vi "solar Menu (Handle).vi"(5 "Target":string, 6 "Is SOLAR UI? (F)":bool, 7 "SOLAR Refnum":T1, 8 "error in (no error)":errorcluster, 9 "ItemTag":string, 10 "MenuRef":refnum<k9>, 11 "VIRef":refnum<vi>) -> (0 "error out":errorcluster)   [LabVIEW 2018]
doc: "This handles the menu selections for the target."
uses:
  <vilib>/Platform/browser.llb/Open URL in Default Browser (string).vi
  solar_ctl SOLAR UI Panes.ctl
  solar_ctl SOLAR Refnum.ctl
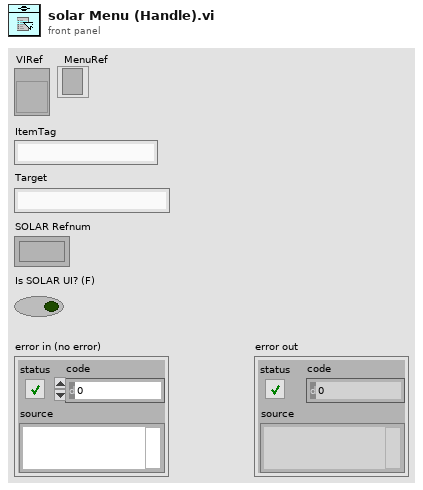
[diagram p1: front panel]
types:
  T1 = typedef "solar_ctl SOLAR Refnum.ctl" = refnum<k1>
  T2 = typedef "solar_ctl SOLAR Global.ctl" = cluster{"Targets":T3[], "AppDir":path, "solar.ini":path, "ConfigsDir":path, "CosmosDir":path, "LogsDir":path, "ExePath":path, "ExeVersion":string, "PartNum":string, "AppSetup":string, "Title":string, "Main.ini":path, "Temp.ini":path, "vSOLAR":string, "Splash.png":string, "SplashWait":i32, "SOLARUE":refnum<user-event>, "VoyagerRefnum":T4, "QTimerRefnum":T5}
  T3 = typedef "solar_ctl Target Global.ctl" = cluster{"Target":string, "Q":refnum<queue>, "UE":refnum<user-event>, "VI":refnum<vi>, "Menu":refnum<k9>, "Data":refnum<data-value>, "Attributes":variant}
  T4 = typedef "solar_voy_ctl Voyager Refnum.ctl" = refnum<k1>
  T5 = typedef "solar_qtimer_ctl Refnum.ctl" = refnum<k1>
  T6 = typedef "solar_ctl SOLAR UI Panes.ctl" = cluster{"Status":bool, "Emergency":bool, "Targets":bool}
  T7 = enum32{"invalid app kind", "Development System", "Run Time System", "Student Edition", "Embedded LabVIEW", "Evaluation", "Custom"}
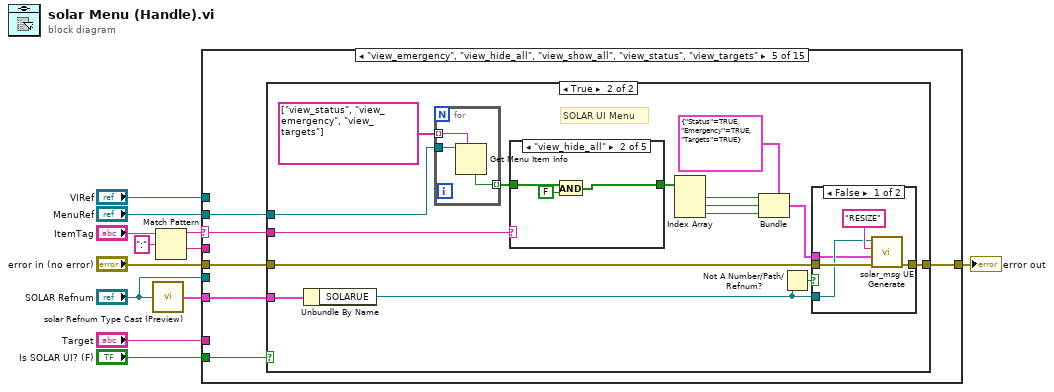
[diagram p0: block diagram]
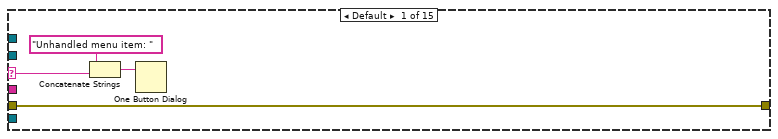
[diagram p2: hidden frame]
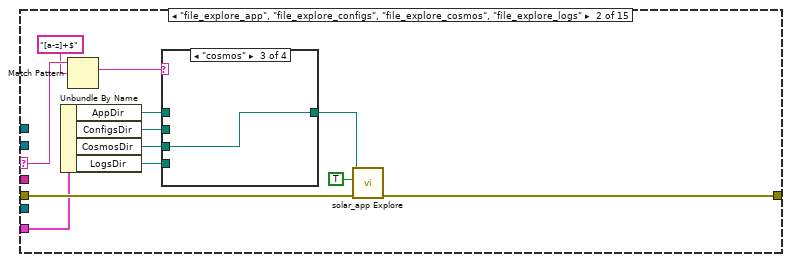
[diagram p3: hidden frame]
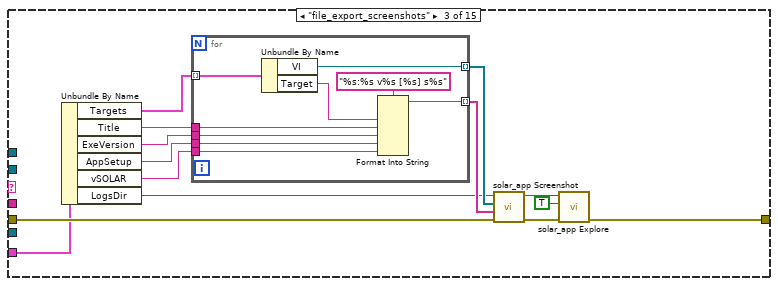
[diagram p7: hidden frame]
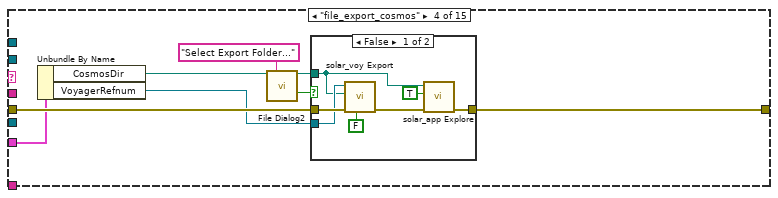
[diagram p8: hidden frame]
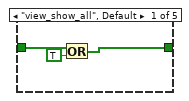
[diagram p11: hidden frame]
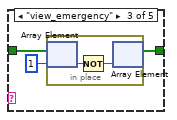
[diagram p12: hidden frame]
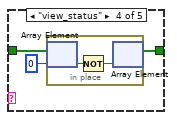
[diagram p13: hidden frame]
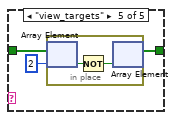
[diagram p14: hidden frame]
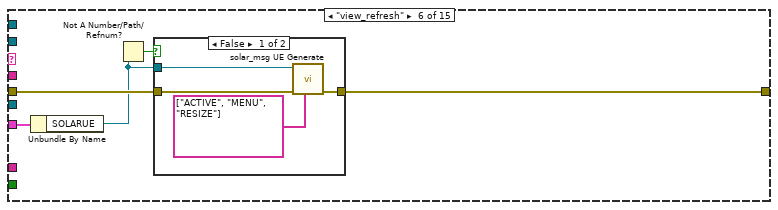
[diagram p16: hidden frame]
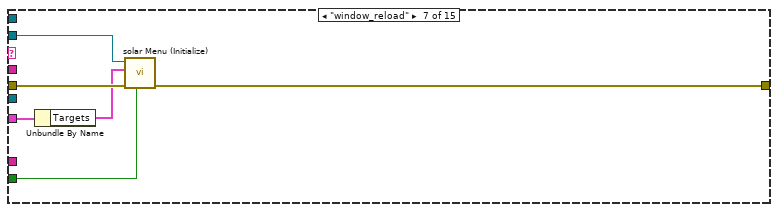
[diagram p18: hidden frame]
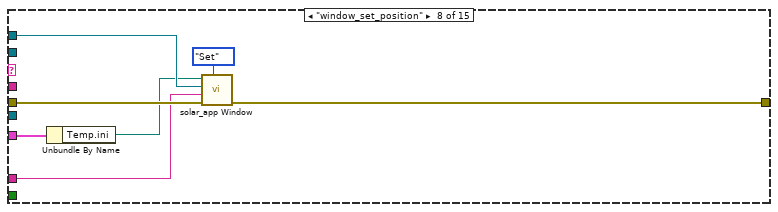
[diagram p19: hidden frame]
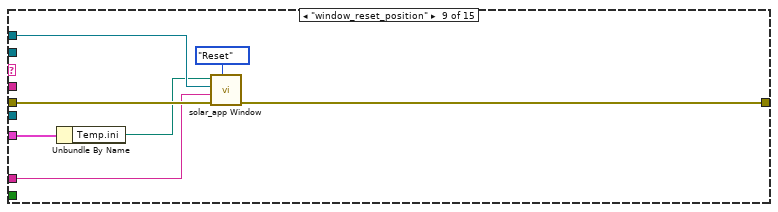
[diagram p20: hidden frame]
diagram:
  n1 = call "solar Refnum Type Cast (Preview).vi"("Refnum"="SOLAR Refnum") -> ("SOLAR"=w2:T2)  [unwired: 8 in]
  n2 = Match Pattern(string="ItemTag", regular expression=":") -> (before substring=w6:string, after substring=w5:string)  [unwired: 1 in, 2 out]
  n3 = case shown="\"view_emergency\", \"view_hide_all\", \"view_show_all\", \"view_status\", \"view_targets\"" w6 {
    selector: w6 -> [w15 w28 _ _ w73 _ _ _ _ _ _ _ _ _ _]
    tunnel: [w16 w24 w42 w63 w77 w128 w139 w143 w150 w157 w167 w185 w187 w211 w213] -> w12
    tunnel: "error in (no error)" -> [w16 w25 w46 w62 w76 w127 w137 w146 w153 w160 w168 w186 w188 w203 w214]
    tunnel: "VIRef" -> [_ _ _ _ _ _ _ w145 w152 w159 _ _ _ _ _]
    tunnel: "MenuRef" -> [_ _ _ _ w74 _ w138 _ _ _ _ _ _ _ _]
    tunnel: w5 -> [_ _ _ _ _ _ _ _ _ _ w166 w184 _ _ _]
    tunnel: "Is SOLAR UI? (F)" -> [_ _ _ _ w72 _ w135 _ _ _ _ _ _ _ _]
    tunnel: w2 -> [_ w21 w34 w57 w75 w125 w136 w141 w148 w155 w164 _ _ w202 _]
    tunnel: "Target" -> [_ _ _ _ _ _ _ w140 w147 w154 _ _ _ _ _]
    tunnel: "SOLAR Refnum" -> [_ _ _ _ _ _ _ _ _ _ _ w182 _ _ _]
    frame Default {
      n4 = Concatenate Strings("Unhandled menu item: ", w15) -> (w14:string)
      n5 = One Button Dialog(message=w14) -> ()  [unwired: 1 in, 1 out]
    }
    frame "file_explore_app", "file_explore_configs", "file_explore_cosmos", "file_explore_logs" {
      n6 = Unbundle By Name(w21) -> ("AppDir"=w17:path, "ConfigsDir"=w20:path, "CosmosDir"=w19:path, "LogsDir"=w18:path)
      n7 = Match Pattern(string=w28, regular expression="[a-z]+$") -> (match substring=w26:string)  [unwired: 1 in, 3 out]
      n8 = case shown="\"cosmos\"" w26 {
        tunnel: w20 -> [_ w30 _ _]
        tunnel: [w29 w30 w31 w32] -> w23
        tunnel: w19 -> [_ _ w31 _]
        tunnel: w18 -> [_ _ _ w32]
        tunnel: w17 -> [w29 _ _ _]
        frame "app", Default {
        }
        frame "configs" {
        }
        frame "cosmos" {
        }
        frame "logs" {
        }
      }
      n9 = call "solar_app Explore.vi"("error in (no error)"=w25, "Open Folder? (F)"=TRUE, "File or Folder Path"=w23) -> ("error out"=w24:errorcluster)  [unwired: 8 in]
    }
    frame "file_export_screenshots" {
      n10 = Unbundle By Name(w34) -> ("Targets"=w33:T3[], "Title"=w40:string, "ExeVersion"=w39:string, "AppSetup"=w38:string, "vSOLAR"=w37:string, "LogsDir"=w35:path)
      n11 = for {
        tunnel: [w55] -> w45 mode=indexing
        tunnel: w39 -> [w53]
        tunnel: w38 -> [w52]
        tunnel: w37 -> [w51]
        tunnel: w40 -> [w50]
        tunnel: [w48] -> w36 mode=indexing
        tunnel: w33 -> [w47] mode=indexing
        n12 = Unbundle By Name(w47) -> ("VI"=w48:refnum<vi>, "Target"=w49:string)
        n13 = Format Into String(format string="%s:%s v%s [%s] s%s", w49, w50, w53, w52, w51) -> (resulting string=w55:string)  [unwired: 2 in, 1 out]
      }
      n14 = call "solar_app Screenshot.vi"("error in (no error)"=w46, "Additional Info"=w45, "VI Refnums"=w36, "LogsDir"=w35) -> ("error out"=w43:errorcluster, "ExportDir"=w41:path)  [unwired: 5 in, 1 out]
      n15 = call "solar_app Explore.vi"("error in (no error)"=w43, "Open Folder? (F)"=TRUE, "File or Folder Path"=w41) -> ("error out"=w42:errorcluster)  [unwired: 8 in]
    }
    frame "file_export_cosmos" {
      n16 = Unbundle By Name(w57) -> ("CosmosDir"=w58:path, "VoyagerRefnum"=w56:T4)
      n17 = call "File Dialog2"("start path"=w58, "prompt"="Select Export Folder...") -> ("selected path"=w60:path, "cancelled"=w59:bool)  [unwired: 10 in, 2 out]
      n18 = case shown="False" w59 {
        tunnel: [w69 w71] -> w63
        tunnel: w62 -> [w68 w71]
        tunnel: w60 -> [w65 _]
        tunnel: w56 -> [w67 _]
        frame False {
          n19 = call "solar_voy Export.vi"("Suppress Errors? (T)"=FALSE, "error in (no error)"=w68, "COSMOS Root (\"\" = Use Default)"=w65, "Voyager Refnum in"=w67) -> ("error out"=w66:errorcluster)  [unwired: 6 in, 1 out]
          n20 = call "solar_app Explore.vi"("error in (no error)"=w66, "Open Folder? (F)"=TRUE, "File or Folder Path"=w65) -> ("error out"=w69:errorcluster)  [unwired: 8 in]
        }
        frame True {
        }
      }
    }
    frame "view_emergency", "view_hide_all", "view_show_all", "view_status", "view_targets" {
      n21 = case shown="True" w72 {
        tunnel: [w78 w93] -> w77
        tunnel: w76 -> [w78 w92]
        tunnel: w75 -> [_ w90]
        tunnel: w74 -> [_ w88]
        tunnel: w73 -> [_ w85]
        frame False {
          # "Child target menu\n-Do nothing"
        }
        frame True {
          # "SOLAR UI Menu"
          n22 = Unbundle By Name(w90) -> ("SOLARUE"=w89:refnum<user-event>)
          n23 = for {
            tunnel: w88 -> [w117]
            tunnel: string[] ["view_status", "view_emergency", "view_targets"] -> [w116] mode=indexing
            tunnel: [w115] -> w86 mode=indexing
            n24 = Get Menu Item Info(7:w116, 11:w117) -> (4:w115:bool)  [unwired: 1 in, 6 out]
          }
          n25 = case shown="\"view_hide_all\"" w85 {
            tunnel: [w94 w97 w100 w105 w110] -> w84
            tunnel: w86 -> [w96 w99 w102 w107 w112]
            frame "view_show_all", Default {
              n26 = Or(x=w96, y=TRUE) -> (x .or. y?=w94:bool[])
            }
            frame "view_hide_all" {
              n27 = And(x=w99, y=FALSE) -> (x .and. y?=w97:bool[])
            }
            frame "view_emergency" {
              n28 = in-place {
                n29 = in-place-array #1(w102, 1) -> (w104:bool)
                n30 = Not(x=w104) -> (.not. x?=w103:bool)
                n31 = in-place-array #1(w103) -> (w100:bool[])  [unwired: 1 out]
              }
            }
            frame "view_status" {
              n32 = in-place {
                n33 = in-place-array #2(w107, 0) -> (w109:bool)
                n34 = Not(x=w109) -> (.not. x?=w108:bool)
                n35 = in-place-array #2(w108) -> (w105:bool[])  [unwired: 1 out]
              }
            }
            frame "view_targets" {
              n36 = in-place {
                n37 = in-place-array #3(w112, 2) -> (w114:bool)
                n38 = Not(x=w114) -> (.not. x?=w113:bool)
                n39 = in-place-array #3(w113) -> (w110:bool[])  [unwired: 1 out]
              }
            }
          }
          n40 = Index Array(array=w84) -> (element #1=w83:bool, element #2=w82:bool, element #3=w81:bool)  [unwired: 3 in]
          n41 = Bundle(cluster=T6 {"Status"=TRUE, "Emergency"=TRUE, "Targets"=TRUE} ("Panes"), "Status"=w83, "Emergency"=w82, "Targets"=w81) -> (w79:T6)
          n42 = Not A Number/Path/Refnum?(number/path/refnum=w89) -> (NaN/Path/Refnum?=w91:bool)
          n43 = case shown="False" w91 {
            tunnel: [w121 w123] -> w93
            tunnel: w92 -> [w120 w123]
            tunnel: w89 -> [w119 _]
            tunnel: w79 -> [w118 _]
            frame False {
              n44 = call "solar_msg UE Generate.vi"("error in (no error)"=w120, "CMD_DATA (Last)"=w118, "CMD (Last)"="RESIZE" ("Packet"), "UserEvent in"=w119) -> ("error out"=w121:errorcluster)  [unwired: 6 in, 1 out]
            }
            frame True {
            }
          }
        }
      }
    }
    frame "view_refresh" {
      n45 = Unbundle By Name(w125) -> ("SOLARUE"=w124:refnum<user-event>)
      n46 = Not A Number/Path/Refnum?(number/path/refnum=w124) -> (NaN/Path/Refnum?=w126:bool)
      n47 = case shown="False" w126 {
        tunnel: [w132 w133] -> w128
        tunnel: w127 -> [w131 w133]
        tunnel: w124 -> [w130 _]
        frame False {
          n48 = call "solar_msg UE Generate.vi"("CMD (Array)"=string[] ["ACTIVE", "MENU", "RESIZE"], "error in (no error)"=w131, "UserEvent in"=w130) -> ("error out"=w132:errorcluster)  [unwired: 7 in, 1 out]
        }
        frame True {
        }
      }
    }
    frame "window_reload" {
      n49 = Unbundle By Name(w136) -> ("Targets"=w134:T3[])
      n50 = call "solar Menu (Initialize).vi"("Is SOLAR UI? (F)"=w135, "error in (no error)"=w137, "Targets"=w134, "MenuRef (NaN = All Menus)"=w138) -> ("error out"=w139:errorcluster)  [unwired: 7 in]
    }
    frame "window_set_position" {
      n51 = Unbundle By Name(w141) -> ("Temp.ini"=w144:path)
      n52 = call "solar_app Window.vi"("Action (Set)"=enum16{"Set", "Reset", "Clear"}."Set", "error in (no error)"=w146, "Target"=w140, "VI Refnum"=w145, "Config Path (*.ini)"=w144) -> ("error out"=w143:errorcluster)  [unwired: 6 in]
    }
    frame "window_reset_position" {
      n53 = Unbundle By Name(w148) -> ("Temp.ini"=w151:path)
      n54 = call "solar_app Window.vi"("Action (Set)"=enum16{"Set", "Reset", "Clear"}."Reset", "error in (no error)"=w153, "Target"=w147, "VI Refnum"=w152, "Config Path (*.ini)"=w151) -> ("error out"=w150:errorcluster)  [unwired: 6 in]
    }
    frame "window_clear_position" {
      n55 = Unbundle By Name(w155) -> ("Temp.ini"=w158:path)
      n56 = call "solar_app Window.vi"("Action (Set)"=enum16{"Set", "Reset", "Clear"}."Clear", "error in (no error)"=w160, "Target"=w154, "VI Refnum"=w159, "Config Path (*.ini)"=w158) -> ("error out"=w157:errorcluster)  [unwired: 6 in]
    }
    frame "window" {
      n57 = Unbundle By Name(w164) -> ("SOLARUE"=w163:refnum<user-event>, "Targets"=w161:T3[], "Temp.ini"=w162:path)
      n58 = Not A Number/Path/Refnum?(number/path/refnum=w163) -> (NaN/Path/Refnum?=w165:bool)
      n59 = case shown="True" w165 {
        tunnel: w168 -> [w173 w179]
        tunnel: [w172 w181] -> w167
        tunnel: w166 -> [w170 w175]
        tunnel: w163 -> [w169 _]
        tunnel: w162 -> [_ w180]
        tunnel: w161 -> [_ w174]
        frame False {
          # "Send Unpin command to SOLAR UI"
          n60 = call "solar_msg UE Generate.vi"("error in (no error)"=w173, "CMD_DATA (Last)"=w170, "CMD (Last)"="UNPIN" ("Packet"), "UserEvent in"=w169) -> ("error out"=w172:errorcluster)  [unwired: 6 in, 1 out]
        }
        frame True {
          # "Invalid SOLAR UI - Open VI Manually"
          n61 = call "solar_ui Unpin.vi"("error in (no error)"=w179, "Target"=w175, "Targets"=w174) -> ("error out"=w178:errorcluster, "VI Refnum"=w177:refnum<vi>)  [unwired: 6 in, 1 out]
          n62 = call "solar_app Window.vi"("Action (Set)"=enum16{"Set", "Reset", "Clear"}."Reset", "error in (no error)"=w178, "Target"=w175, "VI Refnum"=w177, "Config Path (*.ini)"=w180) -> ("error out"=w181:errorcluster)  [unwired: 6 in]
        }
      }
    }
    frame "addon" {
      n63 = call "solar_addon.vi"("Action (Launch)"=enum8{"Launch", "Initialize", "Shutdown"}."Launch", "error in (no error)"=w186, "SOLAR Refnum"=w182, "Launch Addon VI"=w184) -> ("error out"=w185:errorcluster)  [unwired: 6 in, 1 out]
    }
    frame "tools_new_addon" {
      n64 = property class="App"() -> ("App.Kind"=w189:T7)  [unwired: 2 in, 2 out]
      n65 = case shown="Default" w189 {
        tunnel: w188 -> [w190 w200]
        tunnel: [w190 w199] -> w187
        frame "Run Time System" {
          n66 = One Button Dialog(message="Cannot create addon in Run Time System") -> ()  [unwired: 1 in, 1 out]
        }
        frame Default {
          n67 = vi-ref "solar_addon Template.vit"() -> (w193:refnum<vi>)
          n68 = property class="VI (strict)"(reference=w193) -> ("Name"=w192:string)  [unwired: 1 in, 2 out]
          n69 = Open VI Reference(vi path=w192) -> (vi reference=w197:refnum<vi>, error out=w198:errorcluster)  [unwired: 5 in]
          n70 = invoke class="VI" method="FP.Open"(reference=w197, error in=w198) -> (reference out=w195:refnum<vi>, error out=w196:errorcluster)  [unwired: 3 in, 3 out]
          n71 = Close Reference(reference=w195, error in (no error)=w196) -> (error out=w194:errorcluster)
          n72 = Merge Errors(w200, w194) -> (w199:errorcluster)
        }
      }
    }
    frame "help_about" {
      n73 = Unbundle By Name(w202) -> ("vSOLAR"=w206:string, "Splash.png"=w210:string, "ExeVersion"=w209:string, "PartNum"=w208:string, "AppSetup"=w207:string)
      n74 = call "solar_app Splash Open.vi"("App Setup"=w207, "Part Number"=w208, "SOLAR Version"=w206, "error in (no error)"=w203, "Exe Version"=w209, "Splash Path (\"\")"=w210, "Splash msWait (-1)"=-1) -> ("error out"=w205:errorcluster, "Splash VI Refnum"=w204:refnum<vi>)  [unwired: 3 in]
      n75 = call "solar_app Splash Close.vi"("error in (no error)"=w205, "Close Front Panel? (T)"=FALSE, "Splash VI Refnum in"=w204) -> ("error out"=w211:errorcluster)  [unwired: 8 in]
    }
    frame "help_solar" {
      # "Consideration: Pull in from configuration file"
      n76 = VI Library() -> (path=w222:path)
      n77 = Strip Path(path=w222) -> (stripped path=w221:path)  [unwired: 1 out]
      n78 = Build Path(base path=w221, name or relative path=path "help/Ball Aerospace/SOLAR/solar.chm" ("stripped path")) -> (appended path=w215:path)
      n79 = call <vilib>:"Check if File or Folder Exists.vi"("error in (no error)"=w214, "path"=w215) -> ("error out"=w218:errorcluster, "file or folder exists?"=w217:bool, "dup path"=w219:path)  [unwired: 7 in]
      n80 = case shown="True" w217 {
        tunnel: w219 -> [_ w229]
        tunnel: w218 -> [w225 w227]
        tunnel: "https://srv-svn.aero.ball.com/projects/solar" -> [w224 _]
        tunnel: [w223 w226] -> w213
        frame False {
          n81 = call-poly <vilib>:"Open URL in Default Browser.vi"("error in (no error)"=w225, "URL"=w224) -> ("error out"=w223:errorcluster)  [unwired: 4 in, 1 out]
        }
        frame True {
          n82 = Control Online Help(1:w227, 2:w229, 4:enum16{"Contents", "Key", "Close"}."Contents" ("Operation")) -> (0:w226:errorcluster)  [unwired: 1 in]
        }
      }
    }
  }
  "error out" <- w12
